vi "Enable OutPut SDS State.vi"(7 "Channel":i32(ring)=1 items=["Channel 1"=1, "Channel 2"=2, "Channel 3"=3, "Channel 4"=4, "Channel 5"=5, "Channel 6"=6, "Channel 7"=7, "Channel 8"=8, "Channel 8"=9, "Channel 10"=10, "Channel 11"=11, "Channel 12"=12, "Channel 13"=13, "Channel 14"=14, "Channel 15"=15, "Channel 16"=16], 8 "error in":errorcluster, 9 "State":bool, 11 "VISA resource name":refnum<visa-resource-name>) -> (0 "error out":errorcluster, 3 "VISA resource name out":refnum<visa-resource-name>)   [LabVIEW 2020, in "IT-M3400.lvlib"]
doc: "This command is used to set the SDS function state.\n<b>State</b>\n0:Close the SDS State\n1:Open the SDS state"
uses:
  IT-M3400.lvlib
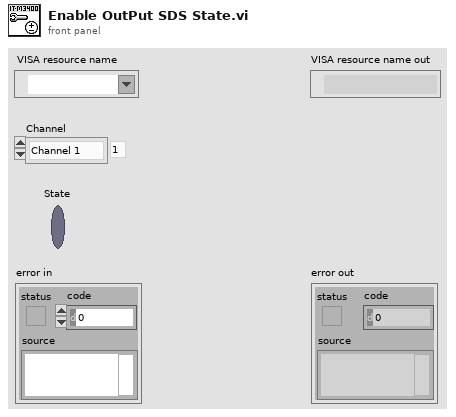
[diagram p1: front panel]
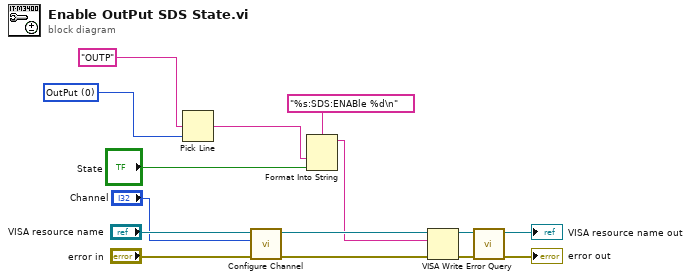
[diagram p0: block diagram]
diagram:
  w4 = u16 0 items=["OutPut"] ("Input&Output(0:Input)")
  n1 = Pick Line(multi-line string="OUTP", line index=w4) -> (output string=w1:string)  [unwired: 1 in]
  n2 = call "Configure Channel.vi"("error in"="error in", "Channel"="Channel", "VISA resource name"="VISA resource name") -> ("error out"=w7:errorcluster, "VISA resource name out"=w8:refnum<visa-resource-name>)  [unwired: 7 in]
  n3 = Format Into String(format string="%s:SDS:ENABle %d\n", w1, "State") -> (resulting string=w5:string)  [unwired: 2 in, 1 out]
  n4 = VISA Write(VISA resource name=w8, write buffer=w5, error in (no error)=w7) -> (VISA resource name out=w12:refnum<visa-resource-name>, error out=w13:errorcluster)  [unwired: 1 out]
  n5 = call "Error Query.vi"("error in"=w13, "VISA resource name"=w12) -> ("error out"=→"error out":errorcluster, "VISA resource name out"=→"VISA resource name out":refnum<visa-resource-name>)  [unwired: 7 in, 1 out]
